vi "Triax320 GetTurretPos.vi"(8 "error in (no error)":errorcluster, 11 "Triax VISA Rsrc":refnum<visa-resource-name>="SR530") -> (0 "error out":errorcluster, 2 "Grating":u8(ring) items=["1", "2", "3"], 3 "Triax VISA Rsrc Out":refnum<visa-resource-name>="SR530")   [LabVIEW 2019]
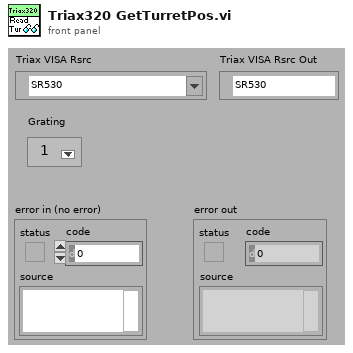
[diagram p1: front panel]
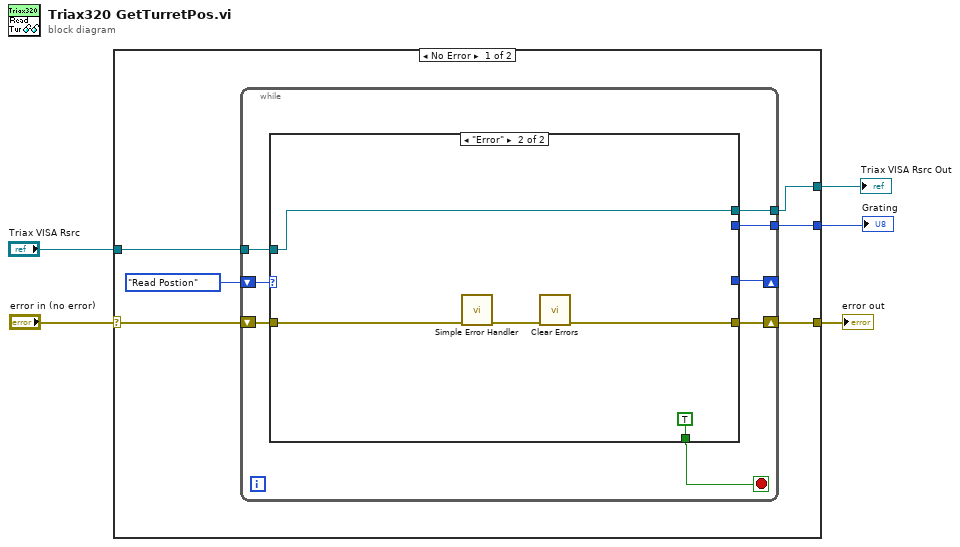
[diagram p0: block diagram]
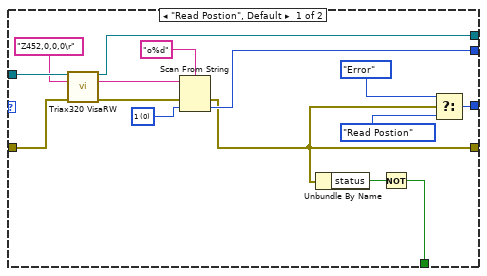
[diagram p2: hidden frame]
diagram:
  n1 = case shown="No Error" "error in (no error)" {
    selector: "error in (no error)" -> [w10 w41]
    tunnel: "Triax VISA Rsrc" -> [w11 w40]
    tunnel: [w8 w41] -> w3
    tunnel: [w7 _] -> w1
    tunnel: [w6 w40] -> w2
    frame No Error {
      n2 = while {
        shift-right: [w17] -> _
        shift-left: enum16{"Error", "Read Postion"}."Read Postion" -> [w19]
        tunnel: w11 -> [w16]
        shift-right: [w14] -> w8
        shift-left: w10 -> [w15]
        tunnel: [w13] -> w6
        tunnel: [w12] -> w7
        stop <- w18 stop-if-true
        n3 = case shown="\"Error\"" w19 {
          tunnel: [w21 TRUE] -> w18
          tunnel: [w30 _] -> w17
          tunnel: w16 -> [w34 w39]
          tunnel: w15 -> [w33 w37]
          tunnel: [w23 w35] -> w14
          tunnel: [w32 w39] -> w13
          tunnel: [w27 _] -> w12
          frame "Read Postion", Default {
            w20 = u8 0 items=["1", "2", "3"] ("Grating")
            n4 = call <userlib>:"Triax320 VisaRW.vi"("VISA Rsrc"=w34, "ChaineCom"="Z452,0,0,0\r" ("chaîne"), "error in (no error)"=w33) -> ("VISA Rsrc Out"=w32:refnum<visa-resource-name>, "ChaineRep"=w29:string, "error out"=w26:errorcluster)  [unwired: 7 in, 3 out]
            n5 = Scan From String(format string="o%d" ("chaîne de format"), input string=w29, error in=w26, default 1=w20) -> (error out=w23:errorcluster, output 1=w27:u8)  [unwired: 1 in, 2 out]
            n6 = Unbundle By Name(w23) -> ("status"=w22:bool)
            n7 = Not(x=w22) -> (.not. x?=w21:bool)
            n8 = Select(t=enum16{"Error", "Read Postion"}."Error", s=w23, f=enum16{"Error", "Read Postion"}."Read Postion") -> (s? t:f=w30:enum16{"Error", "Read Postion"})
          }
          frame "Error" {
            n9 = call <vilib>:"Simple Error Handler.vi"("error in (no error)"=w37) -> ("error out"=w36:errorcluster)  [unwired: 4 in, 4 out]
            n10 = call <vilib>:"Clear Errors.vi"("error in (no error)"=w36) -> ("error out"=w35:errorcluster)  [unwired: 5 in, 1 out]
          }
        }
      }
    }
    frame Error {
    }
  }
  "error out" <- w3
  "Triax VISA Rsrc Out" <- w2
  "Grating" <- w1
